vi "DiscreteIntegrator1_v2_subvi.vi"(6 "Loop Iteration":i32, 9 "IC":dbl, 10 "Time Step":dbl, 11 "Data in":dbl) -> (3 "Integ. Signal":dbl)   [LabVIEW 2019]
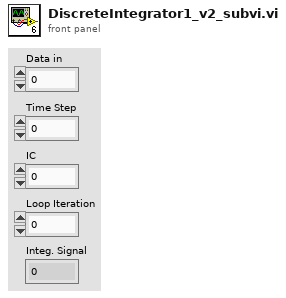
[diagram p1: front panel]
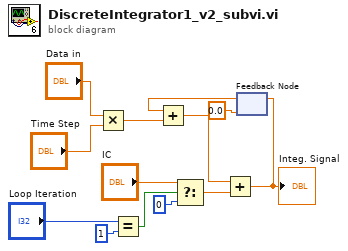
[diagram p0: block diagram]
diagram:
  n1 = Multiply(x="Data in", y="Time Step") -> (x*y=w8:dbl)
  n2 = Equal?(x="Loop Iteration", y=1) -> (x = y?=w4:bool)
  n3 = Select(t="IC", s=w4, f=0) -> (s? t:f=w13:dbl)
  n4 = feedback #1(0.0 ("y")) -> (w10:dbl)
  n5 = Add(x=w10, y=w8) -> (x+y=w11:dbl)
  n6 = Add(x=w11, y=w13) -> (x+y=w12:dbl)
  "Integ. Signal" <- w12
  n7 = feedback-in #1(w12) -> ()
